vi "Unsubscribe.vi"(8 "error in (no error)":errorcluster, 9 "Unique Subscriber ID":string, 10 "Subscription Name":string, 11 "Mediator In":refnum<class "Mediator.lvclass">) -> (0 "error out":errorcluster, 3 "Mediator Out":refnum<class "Mediator.lvclass">)   [LabVIEW 2015, in "Mediator.lvlib" / "Mediator.lvclass"]
uses:
  Mediator.lvclass
panel:
  # "STUB"
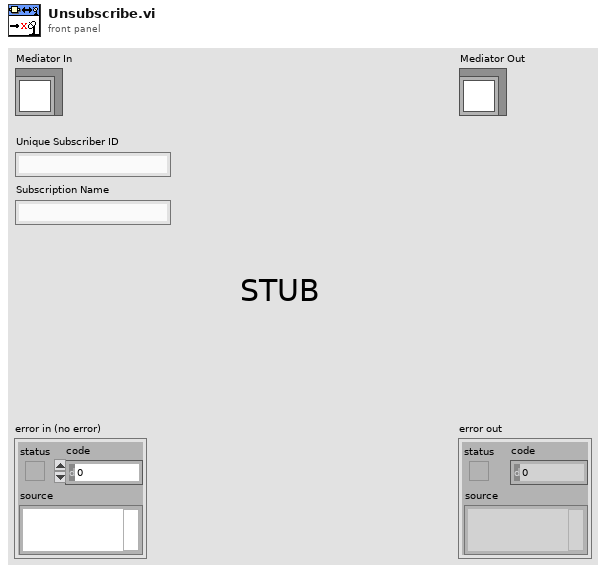
[diagram p1: front panel]
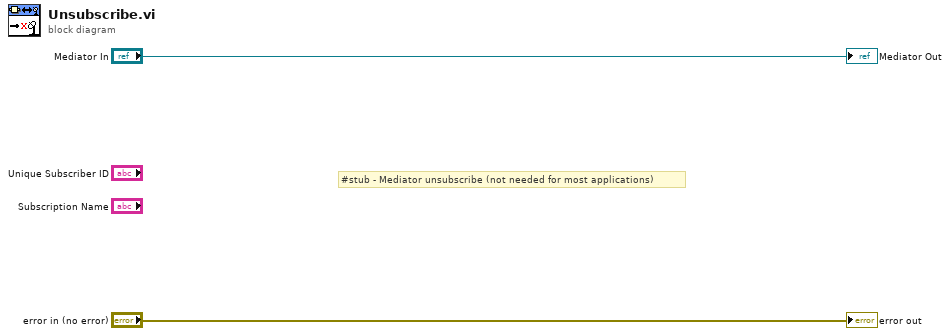
[diagram p0: block diagram]
diagram:
  # "#stub - Mediator unsubscribe (not needed for most applications)"
  "error out" <- "error in (no error)"
  "Mediator Out" <- "Mediator In"
